vi "retrievePythonVersion.vi"(8 "error in (no error)":errorcluster) -> (0 "error out":errorcluster, 2 "Python version":string)   [LabVIEW 2016]
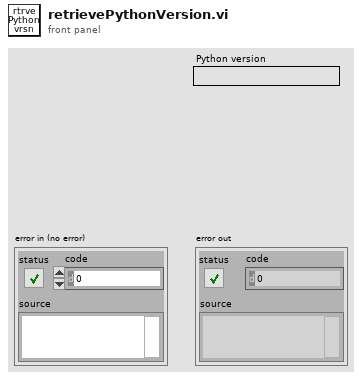
[diagram p1: front panel]
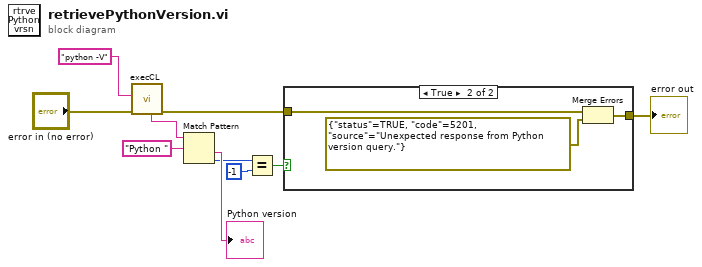
[diagram p0: block diagram]
diagram:
  n1 = call "execCL.vi"("error in (no error)"="error in (no error)", "command line"="python -V") -> ("error out"=w3:errorcluster, "standard error"=w1:string)  [unwired: 6 in, 2 out]
  n2 = Match Pattern(string=w1, regular expression="Python ") -> (after substring=→"Python version":string, offset past match=w6:i32)  [unwired: 1 in, 2 out]
  n3 = Equal?(x=w6, y=-1) -> (x = y?=w4:bool)
  n4 = case shown="True" w4 {
    tunnel: w3 -> [w11 w14]
    tunnel: [w11 w12] -> w2
    frame False {
    }
    frame True {
      n5 = Merge Errors(w14, errorcluster {"status"=TRUE, "code"=5201, "source"="Unexpected response from Python version query."} ("error constant")) -> (w12:errorcluster)
    }
  }
  "error out" <- w2
